vi "Write CAN FIFO Direct Dispatch.vi"(6 "FIFO Timestamps":T1, 8 "error in (no error)":errorcluster, 9 "Timeout (ms)":i32, 10 "Data":T2[](array[typedef]) {"Tags" format="%.0x"; "payload" format="%x"; "identifier" format="%x"}, 11 "CIFTag in":refnum<class "CIFChannels.lvclass">) -> (0 "error out":errorcluster, 1 "timed out?":bool, 3 "CIFTag out":refnum<class "CIF_NIChn_FifoCAN.lvclass">)   [LabVIEW 2021, in "CIF_NIChn_FifoCAN.lvclass"]
uses:
  CIF_NIChn_FifoCAN.lvclass
  D:/dev/CIF-LVCore/src/Channels/CIF_NIChn/NIChn/CIF_NIChn.lvclass
  CIFChannels/CIFChannels.lvclass
  ChannelCommon/typedef/Datatype CAN.ctl
  ChannelCommon/typedef/TimeStamps.ctl
  CIF_NIChn_FifoCAN.lvclass/CIF_NIChn_FifoCAN.ctl
  ChannelCommon/CIFFIFO/CIFfifo.lvclass/CIFfifo.ctl
  NIChn/CIF_NIChn.lvclass/CIF_NIChn.ctl
  ChannelCommon/CIFFIFO/Accessors/Read Length.vi
  <vilib>/CIFChannels/SubVIs/Get dll Path.vi
  ChannelCommon/CIFFIFO/Utilities/Update Header.vi
  ChannelCommon/CIFFIFO/Flatten/CAN Flatten.vi
  ChannelCommon/CIFFIFO/Accessors/Write T0.vi
  ChannelCommon/CIFFIFO/Accessors/Write T_Out.vi
  ChannelCommon/CIFFIFO/Accessors/Write ClockID.vi
  <vilib>/CIF Foundation/CIF Utilities/Time/System Time/Get System Time.vi
  ChannelCommon/Utilities/Flatten Header.vi
  ChannelCommon/CIFFIFO/Flatten/CAN Flatten.vi/be899675-9489-4ae7-9bdb-bbc908cd9623.vi
  ChannelCommon/CIFFIFO/Flatten/CAN Flatten.vi/fa4e04b0-1c28-4039-87e0-9391600efeb5.vi
  ChannelCommon/CIFFIFO/Flatten/CAN Flatten.vi/24dfac9c-4f7b-471b-adb6-3e40fb284e05.vi
  ChannelCommon/CIFFIFO/Accessors/Write Payload Length.vi
  ChannelCommon/CIFFIFO/Accessors/Read Header.vi
  <vilib>/CIF Foundation/CIF Utilities/Time/System Time/LabVIEW Time to TAI Time.vi
  CIFCore/Common/Utilities/Add Error.vi
  ChannelCommon/CIFFIFO/Flatten/CAN Flatten.vi/be899675-9489-4ae7-9bdb-bbc908cd9623.vi/c28b0ead-42ad-4072-80a2-aca7f2bd7ce3.vi
  ChannelCommon/CIFFIFO/Flatten/CAN Flatten.vi/fa4e04b0-1c28-4039-87e0-9391600efeb5.vi/c28b0ead-42ad-4072-80a2-aca7f2bd7ce3.vi
  ChannelCommon/CIFFIFO/Flatten/CAN Flatten.vi/24dfac9c-4f7b-471b-adb6-3e40fb284e05.vi/c28b0ead-42ad-4072-80a2-aca7f2bd7ce3.vi
  <vilib>/CIF Foundation/CIF Utilities/Errors/Append Error Location.vi
  NIChn/CIF_NIChn.lvclass
  <vilib>/CIFChannels/CIFChannelCore.lvlib
  ChannelCommon/CIFFIFO/CIFfifo.lvclass
  ChannelCommon/ChannelCommon.lvlib
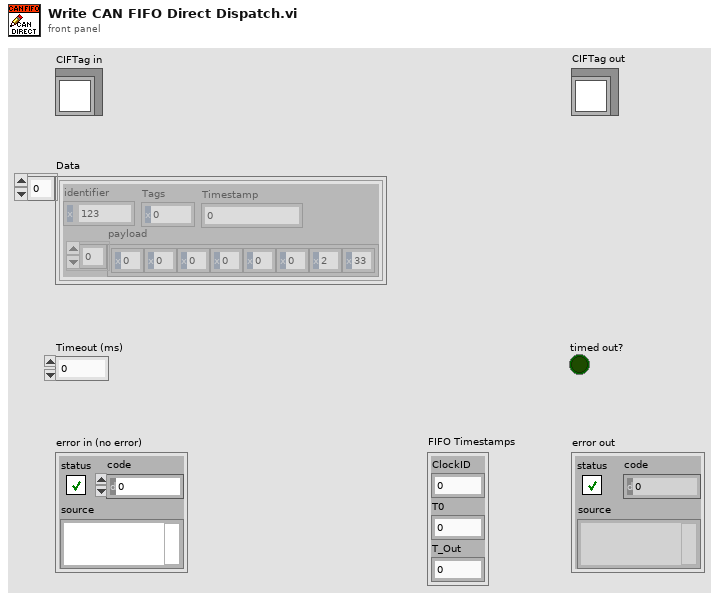
[diagram p1: front panel]
types:
  T1 = typedef "ChannelCommon.lvlib/TimeStamps.ctl" = cluster{"ClockID":u8, "T0":i64, "T_Out":i64}
  T2 = typedef "ChannelCommon.lvlib/Datatype CAN.ctl" = cluster{"payload":u8[], "identifier":u32, "Tags":u8, "Timestamp":u64}
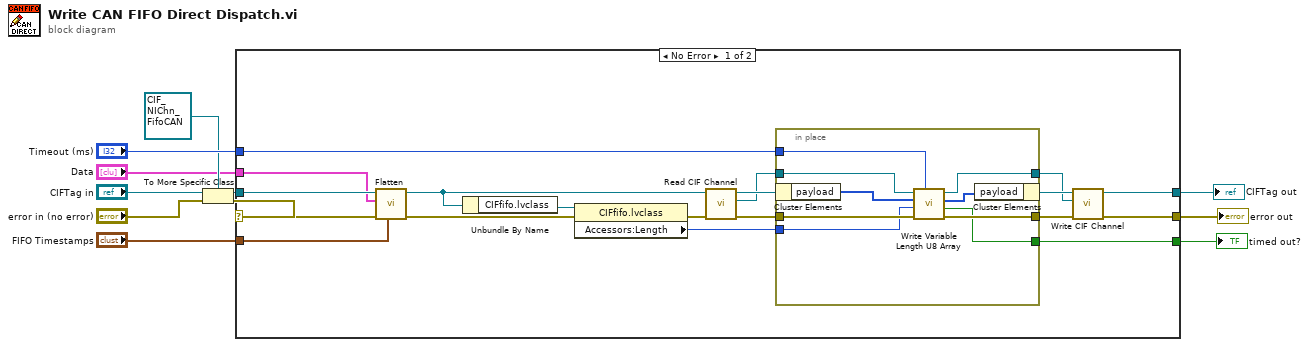
[diagram p0: block diagram]
diagram:
  n1 = To More Specific Class(target class=refnum<class "CIF_NIChn_FifoCAN.lvclass"> refnum ("CIFTag in"), reference="CIFTag in", error in="error in (no error)") -> (specific class reference=w5:refnum<class "CIF_NIChn_FifoCAN.lvclass">, error out=w3:errorcluster)
  n2 = case shown="No Error" w3 {
    selector: w3 -> [w14 w41]
    tunnel: [w21 w41] -> w11
    tunnel: [w26 w40] -> w10
    tunnel: w5 -> [w18 w40]
    tunnel: [w30 _] -> w9
    tunnel: "Timeout (ms)" -> [w22 _]
    tunnel: "Data" -> [w15 _]
    tunnel: "FIFO Timestamps" -> [w12 _]
    frame No Error {
      n3 = call "Flatten.vi"("FIFO Timestamps"=w12, "error in (no error)"=w14, "Data in"=w15, "CIFTag in"=w18) -> ("error out"=w16:errorcluster, "CIFTag out"=w17:refnum<class "CIF_NIChn_FifoCAN.lvclass">)  [unwired: 5 in, 1 out]
      n4 = Unbundle By Name(w17) -> ("CIFfifo.lvclass"=w20:refnum<class "CIFfifo.lvclass">)
      n5 = property class="CIFfifo.lvclass"(reference=w20, error in=w16) -> (error out=w19:errorcluster, "Accessors:Length"=w13:u64)  [unwired: 1 out]
      n6 = call "Read CIF Channel.vi"("error in (no error)"=w19, "CIFTag in"=w17) -> ("error out"=w28:errorcluster, "CIF Channel"=w24:refnum<k21>, "CIFTag out"=w29:refnum<class "CIF_NIChn_FifoCAN.lvclass">)  [unwired: 7 in]
      n7 = in-place {
        in-place-border: w28 -> [w39]
        in-place-border: [w38] -> w25
        in-place-border: [w37] -> w30
        in-place-border: w24 -> [w36]
        in-place-border: [w35] -> w23
        in-place-border: w22 -> [w34]
        in-place-border: w13 -> [w32]
        n8 = in-place-cluster #1(w29) -> ("payload"=w33:u8[])
        n9 = call <vilib>:"Write Variable Length U8 Array.vi"("Timeout (ms)"=w34, "error in"=w39, "numElements"=w32, "U8 Array in"=w33, "CIF Channel in"=w36) -> ("error out"=w38:errorcluster, "Timed out?"=w37:bool, "U8 Array out"=w31:u8[], "CIF Channel out"=w35:refnum<k21>)  [unwired: 3 in]
        n10 = in-place-cluster #1("payload"=w31) -> (w27:refnum<class "CIF_NIChn_FifoCAN.lvclass">)
      }
      n11 = call "Write CIF Channel.vi"("error in (no error)"=w25, "CIF Channel"=w23, "CIFTag in"=w27) -> ("error out"=w21:errorcluster, "CIFTag out"=w26:refnum<class "CIF_NIChn_FifoCAN.lvclass">)  [unwired: 7 in]
    }
    frame Error {
    }
  }
  "error out" <- w11
  "CIFTag out" <- w10
  "timed out?" <- w9
